vi "SetGNSSLogCMD (SubVI).vi"(0 "VISA":refnum<visa-resource-name>, 1 "GNSSLogCMD":string, 3 "error in":errorcluster) -> (7 "VISA out":refnum<visa-resource-name>, 10 "error out":errorcluster)   [LabVIEW 2019]
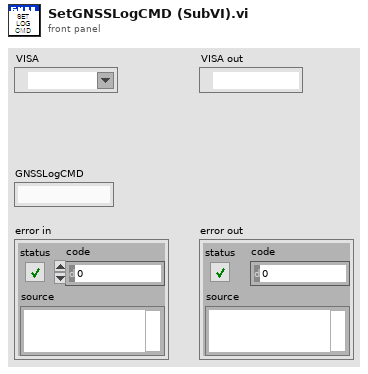
[diagram p1: front panel]
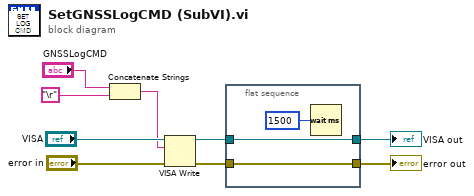
[diagram p0: block diagram]
diagram:
  n1 = Concatenate Strings("GNSSLogCMD", "\r") -> (w3:string)
  n2 = VISA Write(VISA resource name="VISA", write buffer=w3, error in (no error)="error in") -> (VISA resource name out=w8:refnum<visa-resource-name>, error out=w9:errorcluster)  [unwired: 1 out]
  n3 = flat-sequence {
    tunnel: [w11] -> w4
    tunnel: w8 -> [w11]
    tunnel: w9 -> [w10]
    tunnel: [w10] -> w5
    frame #0 {
      n4 = Wait (ms)(milliseconds to wait=u32 1500) -> ()  [unwired: 1 out]
    }
  }
  "error out" <- w5
  "VISA out" <- w4
